vi "test_riccat_02Ni.vi"() -> (3 "All Tests Passed":bool)   [LabVIEW 2019]
uses:
  <vilib>/Analysis/Matrix/Datatypes/RealMatrix.ctl
  <vilib>/Rock Robotics/WPI/ThirdParty/JAS_Junk/TrajLib/Trajectory_Library.lvlib
  <vilib>/Analysis/Matrix/NI_Matrix.lvlib
panel:
  out "R1":T1
  out "Q1":T1
  out "N1":T1
  out "Make N Good":bool
  in  "AREF":T1=[[0.5, 1.0], [0.0, 1.0]]
  out "error out 2":errorcluster
  out "Pos Semi Definite":bool
  out "Q_Chk_Passed":bool
  out "C":T1
  out "Q Check":T1
  out "Bad":bool
  out "Stable Bad":bool
  out "error out":errorcluster
  out "Eigenvalues":cdb[](array[numeric])
  out "Error":bool
  out "Iterations":i32
  out "Elapsed \nTime MS":dbl
  out "ZERO":T1
  out "X  Answer":T1
  in  "R":T1=[[0.3]]
  in  "Q":T1=[[1.0, 0.0], [0.0, 0.0]]
  in  "B":T1=[[0.0], [1.0]]
  in  "A":T1=[[1.0, 1.0], [0.0, 1.0]]
  # "// ------------------------------------------------------------\n  // Test 2: invertible A"
  # "A2 << \n             1, 1, \n              0, 1;"
  # "B2 << \n        0, \n        1;"
  # "Solution weight ??"
  # "Q2 << \n         1, 0, \n         0, 0;"
  # "Example G2"
  # "Cost ??"
  # "R2 << 0.3;"
  # "0.5, 1, \n0, 1;"
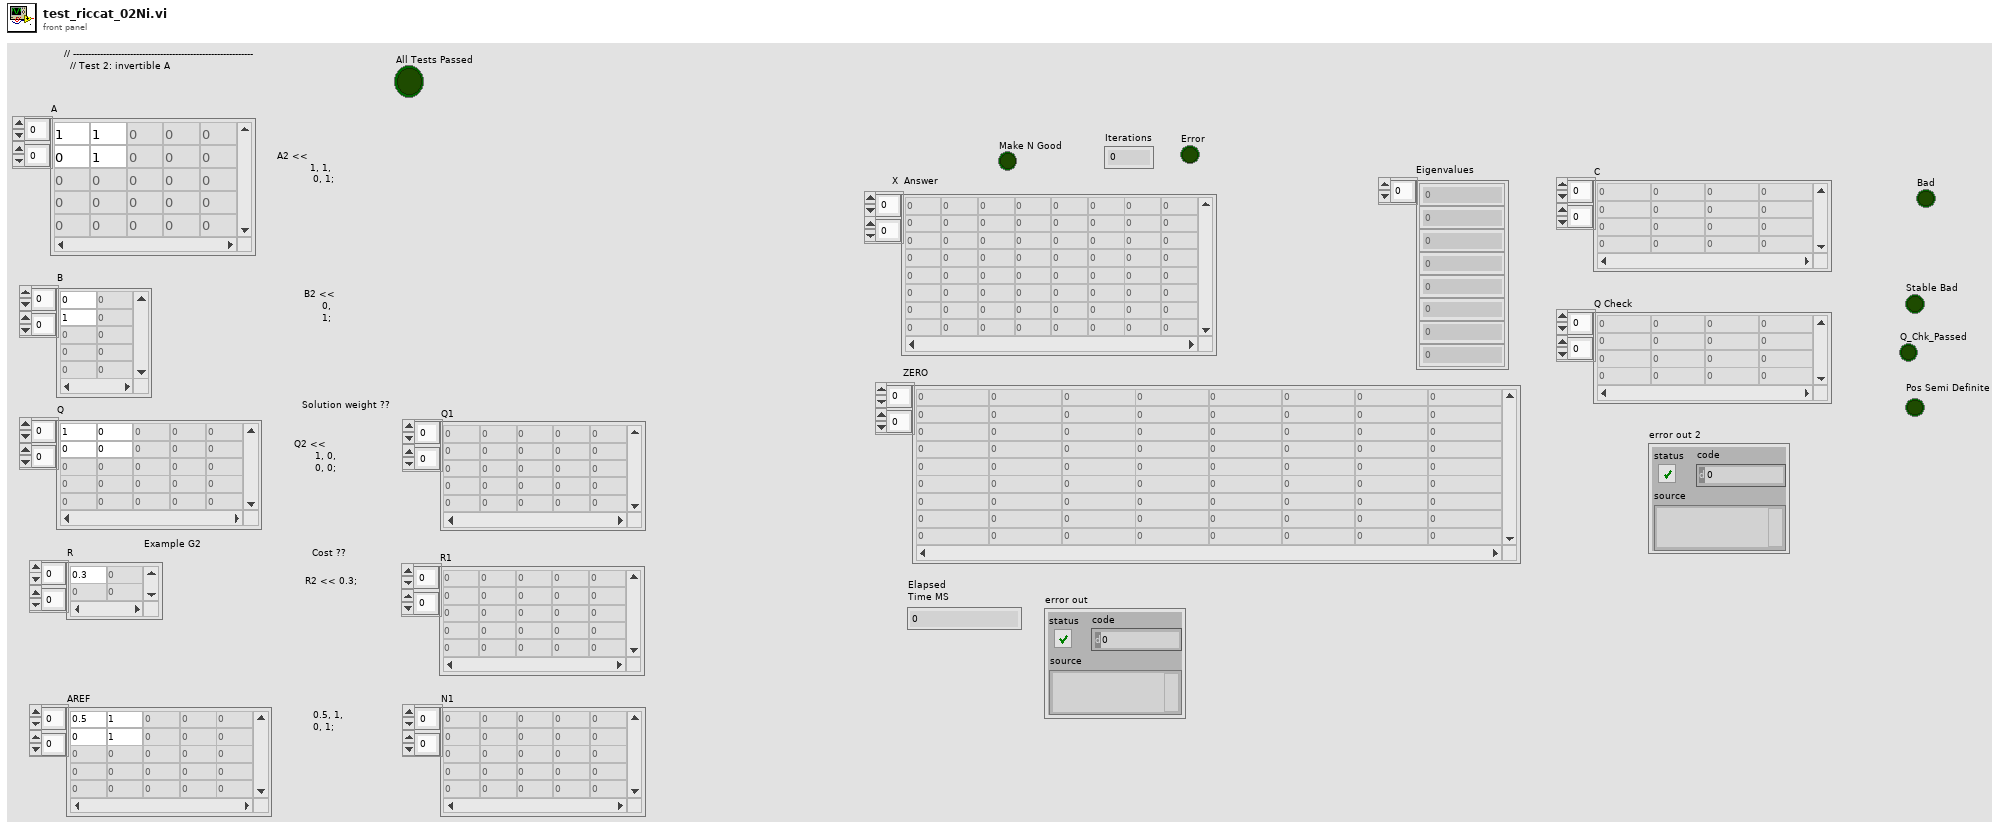
[diagram p1: front panel]
types:
  T1 = typedef "NI_Matrix.lvlib/RealMatrix.ctl" = dbl[][]
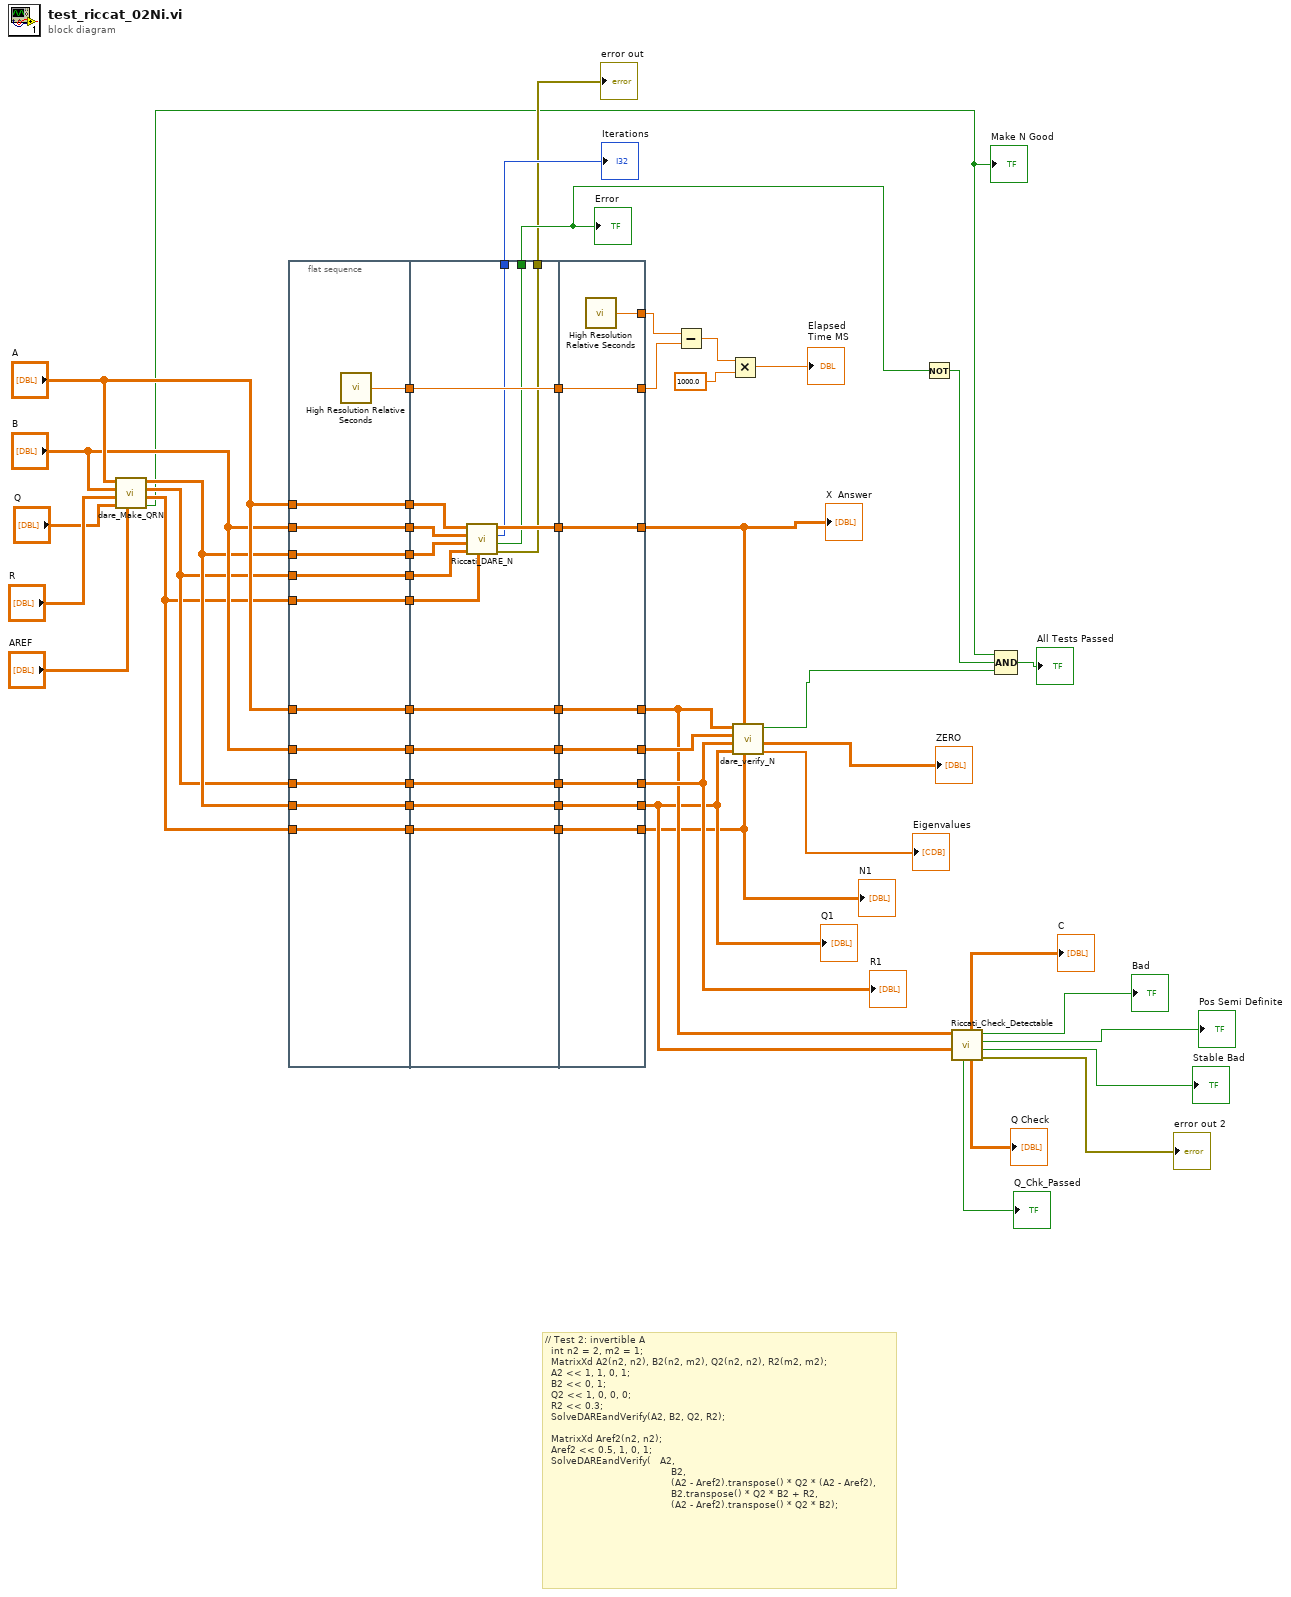
[diagram p0: block diagram]
diagram:
  # "// Test 2: invertible A\n  int n2 = 2, m2 = 1;\n  MatrixXd A2(n2, n2), B2(n2, m2), Q2(n2, n2), R2(m2, m2);\n  A2 << 1, 1, 0, 1;\n  B2 << 0, 1;\n  Q2 << 1, 0, 0, 0;\n  R2 << 0.3;\n  SolveDAREandVerify(A2, B2, Q2, R2);\n\n  MatrixXd Aref2(n2, n2);\n  Aref2 << 0.5, 1, 0, 1;\n  SolveDAREandVerify(   A2, \n                                          B2, \n                                          (A2 - Aref2).transpose() * Q2 * (A2 - Aref2),\n                                          B2.transpose() * Q2 * B2 + R2, \n                                          (A2 - Aref2).transpose() * Q2 * B2);"
  n1 = call "dare_Make_QRN.vi"("AREF"="AREF", "Q"="Q", "R"="R", "B"="B", "A"="A") -> ("Good"=w2:bool, "N1"=w6:T1, "R1"=w8:T1, "Q1"=w9:T1)  [unwired: 3 in]
  "Make N Good" <- w2
  n2 = flat-sequence {
    tunnel: "B" -> [w59]
    tunnel: "A" -> [w60]
    tunnel: "B" -> [w61]
    tunnel: w9 -> [w62]
    tunnel: "A" -> [w63]
    tunnel: w8 -> [w64]
    tunnel: [w64] -> w53
    tunnel: [w63] -> w52
    tunnel: [w62] -> w51
    tunnel: [w61] -> w50
    tunnel: [w60] -> w49
    tunnel: [w59] -> w48
    tunnel: w8 -> [w58]
    tunnel: [w58] -> w43
    tunnel: w9 -> [w57]
    tunnel: [w57] -> w42
    tunnel: [w56] -> w37
    tunnel: w6 -> [w55]
    tunnel: [w55] -> w7
    tunnel: w6 -> [w54]
    tunnel: [w54] -> w5
    tunnel: w53 -> [w79]
    tunnel: w52 -> [w77]
    tunnel: w51 -> [w76]
    tunnel: w50 -> [w75]
    tunnel: w49 -> [w74]
    tunnel: w48 -> [w73]
    tunnel: [w78] -> w47
    tunnel: [w74] -> w46
    tunnel: [w73] -> w45
    tunnel: [w72] -> w44
    tunnel: w43 -> [w72]
    tunnel: w42 -> [w71]
    tunnel: [w71] -> w41
    tunnel: [w70] -> w38
    tunnel: w37 -> [w70]
    tunnel: [w69] -> w33
    tunnel: [w68] -> w32
    tunnel: [w67] -> w23
    tunnel: w7 -> [w66]
    tunnel: w5 -> [w65]
    tunnel: [w65] -> w4
    tunnel: [w85] -> w30
    tunnel: [w86] -> w19
    tunnel: [w87] -> w31
    tunnel: w47 -> [w87]
    tunnel: w46 -> [w86]
    tunnel: w45 -> [w85]
    tunnel: w44 -> [w81]
    tunnel: [w84] -> w18
    tunnel: w41 -> [w84]
    tunnel: [w83] -> w40
    tunnel: [w82] -> w39
    tunnel: w38 -> [w82]
    tunnel: [w81] -> w29
    tunnel: w4 -> [w80]
    tunnel: [w80] -> w3
    frame #0 {
      n3 = call <vilib>:"High Resolution Relative Seconds.vi"() -> ("relative seconds"=w56:dbl)
    }
    frame #1 {
      n4 = call <vilib>:"Riccati_DARE_N.vi"("N"=w66, "R"=w79, "Q"=w76, "B"=w75, "A"=w77) -> ("error out"=w67:errorcluster, "Error"=w68:bool, "Iterations"=w69:i32, "Answer"=w78:T1)  [unwired: 3 in]
    }
    frame #2 {
      n5 = call <vilib>:"High Resolution Relative Seconds.vi"() -> ("relative seconds"=w83:dbl)
    }
  }
  n6 = Subtract(x=w40, y=w39) -> (x-y=w36:dbl)
  n7 = Multiply(x=w36, y=1000.0) -> (x*y=→"Elapsed \nTime MS":dbl)
  n8 = call "dare_verify_N.vi"("N"=w3, "Answer"=w31, "Q"=w18, "R"=w29, "B"=w30, "A"=w19) -> ("Eigenvalues"=→"Eigenvalues":cdb[], "ZERO"=→"ZERO":T1, "Passed"=w25:bool)  [unwired: 3 in]
  n9 = Not(x=w32) -> (.not. x?=w26:bool)
  n10 = call <vilib>:"Riccati_Check_Detectable.vi"("Q"=w18, "A"=w19) -> ("error out"=→"error out 2":errorcluster, "Stable Bad"=→"Stable Bad":bool, "Pos Semi Definite"=→"Pos Semi Definite":bool, "Bad"=→"Bad":bool, "Q_Check"=→"Q Check":T1, "C"=→"C":T1, "Q_Chk_Passed"=→"Q_Chk_Passed":bool)  [unwired: 3 in]
  n11 = Compound Arithmetic op=AND(w2, w26, w25) -> (→"All Tests Passed":bool)
  "X  Answer" <- w31
  "Iterations" <- w33
  "Error" <- w32
  "error out" <- w23
  "N1" <- w3
  "Q1" <- w18
  "R1" <- w29
